vi "create Timings.vi"(8 "error in (no error)":errorcluster, 10 "Parameters":u32[](array[numeric]), 11 "Burst in":refnum<class "Burst.lvclass">) -> (0 "error out":errorcluster, 1 "wait":i32[](array[numeric])=[0, 30000, 0, 0], 2 "timeout":u32[](array[numeric]), 3 "Burst out":refnum<class "Burst.lvclass">)   [LabVIEW 2013, in "Burst.lvclass"]
uses:
  Burst.lvclass
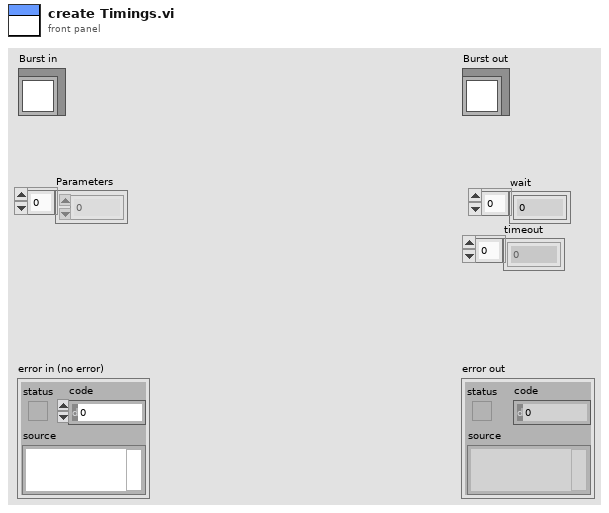
[diagram p1: front panel]
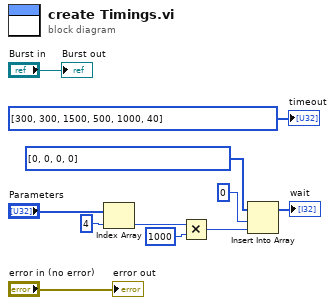
[diagram p0: block diagram]
diagram:
  n1 = Index Array(array="Parameters", index=4) -> (element=w3:u32)
  n2 = Multiply(x=w3, y=u32 1000) -> (x*y=w1:u32)
  n3 = Insert Into Array(array=i32[] [0, 0, 0, 0] ("Timings"), index=0, new element=w1) -> (→"wait":i32[])
  "error out" <- "error in (no error)"
  "Burst out" <- "Burst in"
  "timeout" <- u32[] [300, 300, 1500, 500, 1000, 40] ("Timings")
